vi "Write Error.vi"(2 "error in (no error)":errorcluster, 3 "Plugin Name":string) -> (4 "cleared error":errorcluster)   [LabVIEW 2021, in "CIFLogs.lvlib"]
uses:
  CIFLogs.lvlib
  Typedef/Message Type.ctl
  CIFClocks/Time Conversion/LabVIEW Time to UTC Time.vi
  CIFCore/Common/Utilities/Add Error.vi
  CIFCore/Common/Utilities/Append Error Location.vi
  CIFCore/Common/CIFCoreCommon.lvlib
  CIFClocks/CIFClocks.lvlib
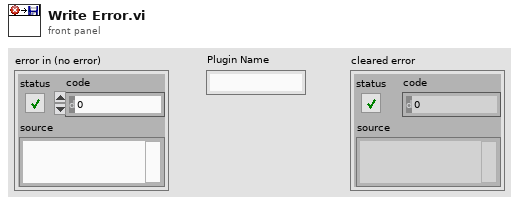
[diagram p1: front panel]
types:
  T1 = typedef "CIFLogs.lvlib/Message Type.ctl" = enum16{"Error", "Information", "Print Terminal", "Configuration"}
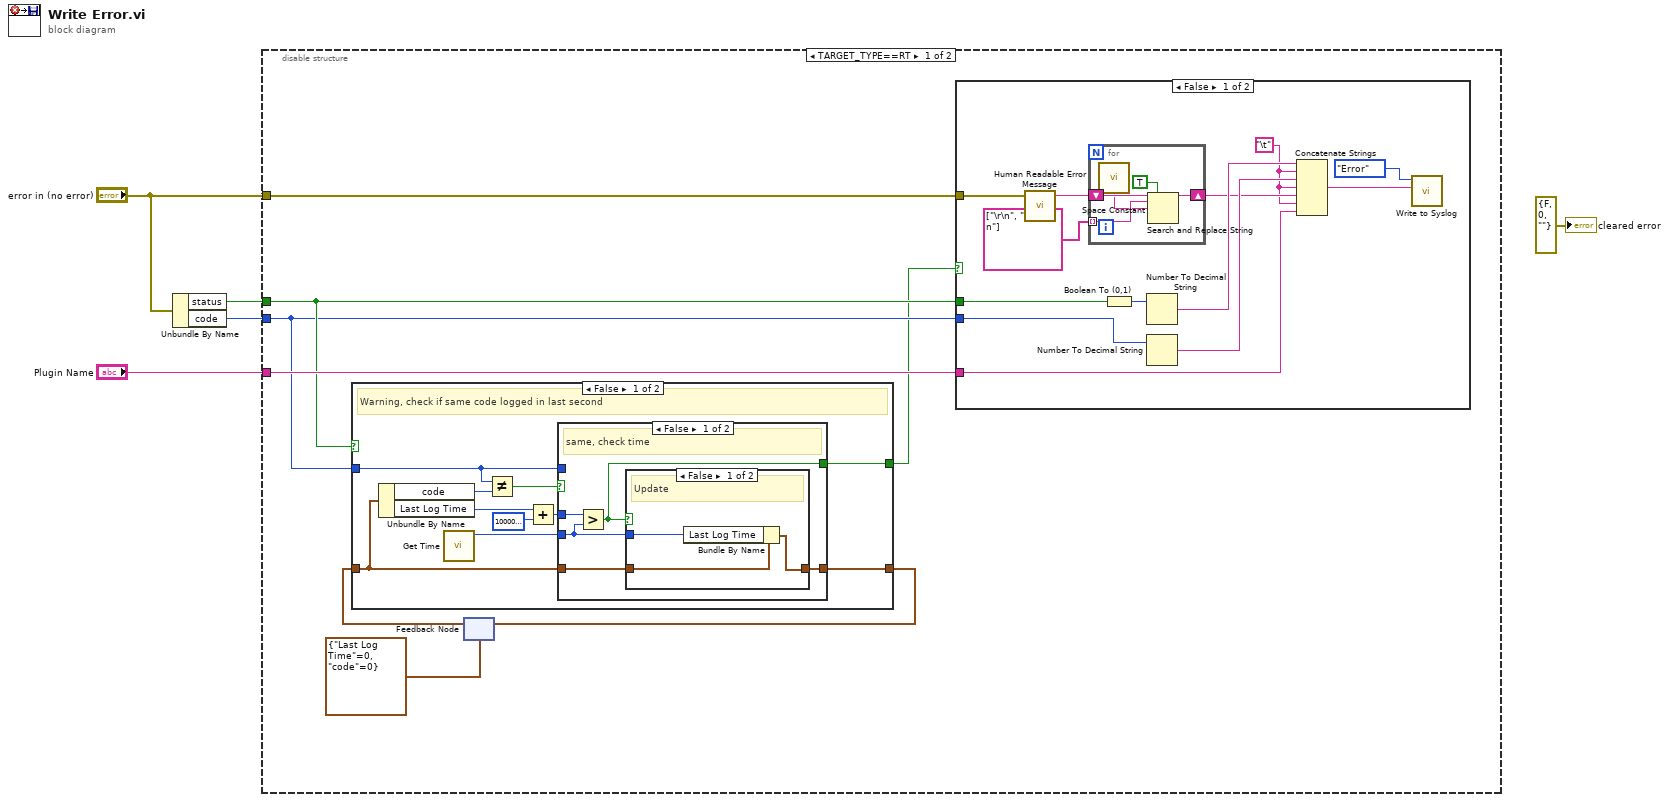
[diagram p0: block diagram]
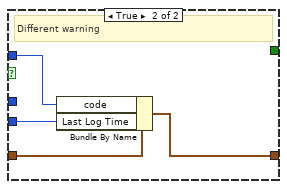
[diagram p3: hidden frame]
diagram:
  n1 = Unbundle By Name("error in (no error)") -> ("status"=w5:bool, "code"=w4:i32)
  n2 = disable-structure shown="TARGET_TYPE==RT" {
    disable-tunnel: w5 -> [w10 _]
    disable-tunnel: w4 -> [w9 _]
    disable-tunnel: "Plugin Name" -> [w13 _]
    disable-tunnel: "error in (no error)" -> [w12 _]
    frame condition #0 (active) {
      n3 = feedback #1(cluster{"Last Log Time":u64, "code":i32} {"Last Log Time"=0, "code"=0}) -> (w8:cluster{"Last Log Time":u64, "code":i32})
      n4 = case shown="False" w10 {
        tunnel: w9 -> [w16 _]
        tunnel: w8 -> [w14 w37]
        tunnel: [w17 _] -> w7
        tunnel: [w15 w37] -> w6
        frame False {
          # "Warning, check if same code logged in last second"
          n5 = Unbundle By Name(w14) -> ("code"=w23:i32, "Last Log Time"=w20:u64)
          n6 = call "Get Time.vi"() -> ("Time (ns)"=w21:u64)  [unwired: 9 in, 2 out]
          n7 = Not Equal?(x=w16, y=w23) -> (x != y?=w22:bool)
          n8 = Add(x=w20, y=u64 1000000000) -> (x+y=w18:u64)
          n9 = case shown="False" w22 {
            tunnel: w21 -> [w24 w36]
            tunnel: w18 -> [w28 _]
            tunnel: [w27 _] -> w17
            tunnel: w16 -> [_ w35]
            tunnel: [w25 w34] -> w15
            tunnel: w14 -> [w26 w33]
            frame False {
              # "same, check time"
              n10 = Greater?(x=w28, y=w24) -> (0:w27:bool)
              n11 = case shown="False" w27 {
                tunnel: w26 -> [w31 w32]
                tunnel: [w30 w32] -> w25
                tunnel: w24 -> [w29 _]
                frame False {
                  # "Update"
                  n12 = Bundle By Name(cluster=w31, "Last Log Time"=w29) -> (w30:cluster{"Last Log Time":u64, "code":i32})
                }
                frame True {
                  # "Skip update"
                }
              }
            }
            frame True {
              # "Different warning"
              n13 = Bundle By Name(cluster=w33, "code"=w35, "Last Log Time"=w36) -> (w34:cluster{"Last Log Time":u64, "code":i32})
            }
          }
        }
        frame True {
          # "Log all Errors"
        }
      }
      n14 = feedback-in #1(w6) -> ()
      n15 = case shown="False" w7 {
        tunnel: w10 -> [w50 _]
        tunnel: w9 -> [w47 _]
        tunnel: w13 -> [w42 _]
        tunnel: w12 -> [w39 _]
        frame False {
          w43 = "\t"
          n16 = call "Human Readable Error Message.vi"("error in (no error)"=w39) -> ("Human readable error message"=w38:string)  [unwired: 4 in]
          n17 = for {
            tunnel: string[] ["\r\n", "\r", "\n"] -> [w54] mode=indexing
            shift-right: [w52] -> w44
            shift-left: w38 -> [w55]
            n18 = call <vilib>:"Space Constant.vi"() -> ("String"=w51:string)
            n19 = Search and Replace String(replace all?=TRUE ("replace all? (F)"), input string=w55, search string=w54, replace string=w51) -> (result string=w52:string)  [unwired: 4 in, 3 out]
          }
          n20 = Boolean To (0,1)(Boolean=w50) -> (0, 1=w48:i16)
          n21 = Number To Decimal String(number=w48) -> (decimal integer string=w46:string)  [unwired: 1 in]
          n22 = Number To Decimal String(number=w47) -> (decimal integer string=w45:string)  [unwired: 1 in]
          n23 = Concatenate Strings(w46, w43, w45, w43, w44, w43, w42) -> (w41:string)
          n24 = call "Write to Syslog.vi"("message"=w41, "CIF Message Type"=Message_Type."Error") -> ()  [unwired: 9 in, 1 out]
        }
        frame True {
          # "Repeating warning, skip log"
        }
      }
    }
    frame condition #1 {
    }
  }
  "cleared error" <- errorcluster {"status"=FALSE, "code"=0, "source"=""} ("cleared error")
